vi "uart.vi"() -> ()   [LabVIEW 2018]
uses:
  <vilib>/Instr/_visa.llb/VISA Configure Serial Port (Instr).vi
panel:
  in  "Characters to Write":string
  out "concatenated string":string
  in  "timeout (10sec)":u32=10000
  in  "stop":bool
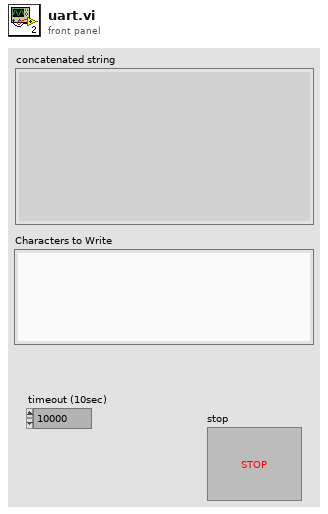
[diagram p1: front panel]
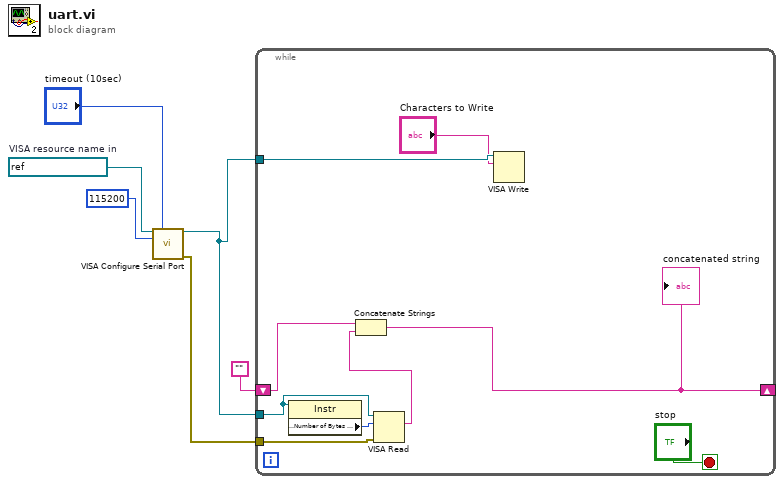
[diagram p0: block diagram]
diagram:
  w6 = refnum<visa-resource-name> "ASRL2::INSTR"  # VISA resource name in
  n1 = call-poly "VISA Configure Serial Port"("VISA resource name"=w6, "timeout (10sec)"="timeout (10sec)", "baud rate (9600)"=u32 115200) -> ("VISA resource name out"=w2:refnum<visa-resource-name>, "error out"=w1:errorcluster)  [unwired: 11 in]
  n2 = while {
    tunnel: w2 -> [w14]
    shift-right: [w11] -> _
    shift-left: "" -> [w12]
    tunnel: w2 -> [w9]
    tunnel: w1 -> [w7]
    stop <- "stop" stop-if-true
    n3 = property class="Instr"(reference=w14) -> ("Serial Settings:Number of Bytes at Serial Port"=w13:u32)  [unwired: 1 in, 2 out]
    n4 = VISA Read(VISA resource name=w14, byte count=w13, error in (no error)=w7) -> (read buffer=w10:string)  [unwired: 3 out]
    n5 = Concatenate Strings(w12, w10) -> (w11:string)
    "concatenated string" <- w11
    n6 = VISA Write(VISA resource name=w9, write buffer="Characters to Write") -> ()  [unwired: 1 in, 3 out]
  }
